vi "Utility_getIterationTime.vi"(2 "Duration (previous)":i64, 3 "End Time (previous)":i64, 4 "Start Time (current)":i64) -> (0 "Time (Sec)":dbl)   [LabVIEW 2009, in "Utility.lvlib"]
doc: "Calculates the time passed from the begining of the previous iteration to the begining of current iteration.\nConnect corresponding inputs from timed loop structure (assumed to use ms in that).\nOutputs the time in seconds."
uses:
  Utility.lvlib
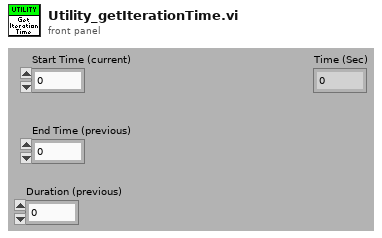
[diagram p1: front panel]
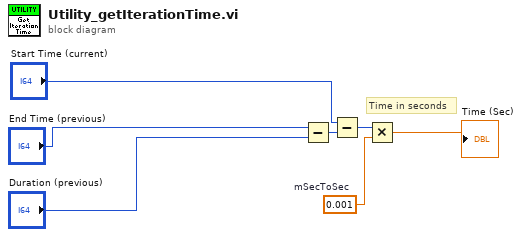
[diagram p0: block diagram]
diagram:
  w5 = 0.001  # mSecToSec
  # "Time in seconds"
  n1 = Subtract(x="End Time (previous)", y="Duration (previous)") -> (x-y=w7:i64)
  n2 = Subtract(x="Start Time (current)", y=w7) -> (x-y=w6:i64)
  n3 = Multiply(x=w6, y=w5) -> (x*y=→"Time (Sec)":dbl)
